vi "Init.vi"(8 "error in (no error)":errorcluster, 11 "XML Report in":refnum<class "XML Report.lvclass">) -> (0 "error out":errorcluster, 3 "XML Report out":refnum<class "XML Report.lvclass">)   [LabVIEW 2020, in "XML Report.lvclass"]
uses:
  XML Report.lvclass
  XML Report.lvclass/XML Report.ctl
  User Interface/Support/Paths.lvlib
  Framework/Configuration Manager/Configuration Manager.lvclass
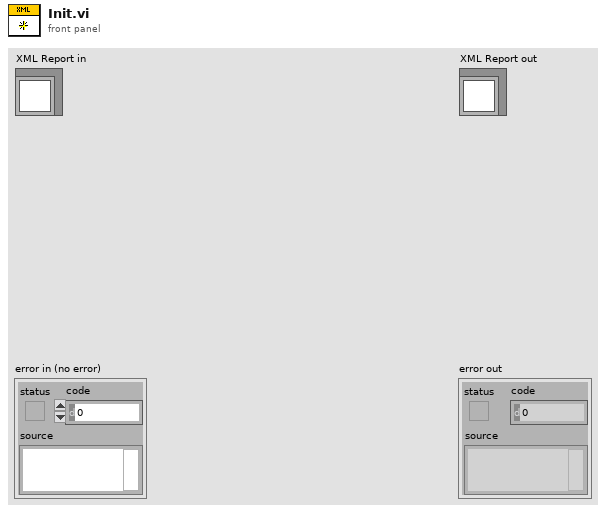
[diagram p1: front panel]
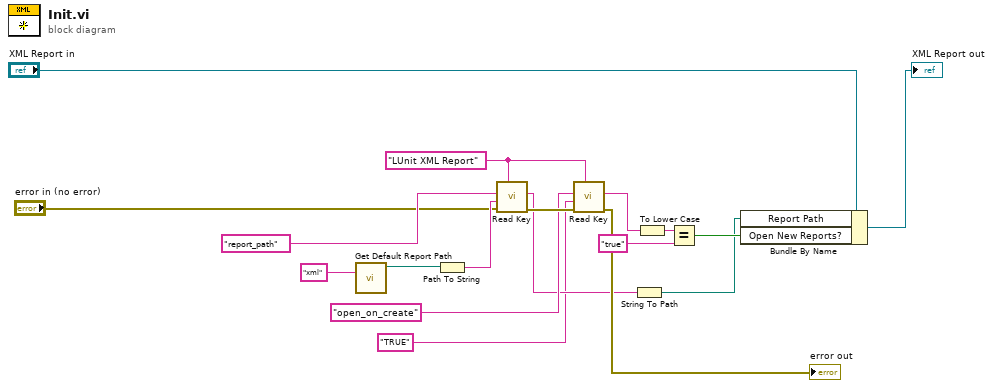
[diagram p0: block diagram]
diagram:
  w10 = "LUnit XML Report"
  n1 = call "Get Default Report Path.vi"("File Extension"="xml") -> ("Default Report Path"=w8:path)  [unwired: 9 in, 1 out]
  n2 = Path To String(path=w8) -> (string=w16:string)
  n3 = call "Read Key.vi"("section"=w10, "error in (no error)"="error in (no error)", "default value"=w16, "key"="report_path" ("Name")) -> ("error out"=w18:errorcluster, "value"=w3:string)  [unwired: 6 in]
  n4 = call "Read Key.vi"("section"=w10, "error in (no error)"=w18, "default value"="TRUE", "key"="open_on_create" ("Name")) -> ("error out"=→"error out":errorcluster, "value"=w13:string)  [unwired: 6 in]
  n5 = String To Path(string=w3) -> (path=w2:path)
  n6 = To Lower Case(string=w13) -> (all lower case string=w12:string)
  n7 = Equal?(x=w12, y="true") -> (x = y?=w4:bool)
  n8 = Bundle By Name(cluster="XML Report in", "Report Path"=w2, "Open New Reports?"=w4) -> (→"XML Report out":refnum<class "XML Report.lvclass">)
